vi "Examples.vi"(6 "Python version":string="3.9", 7 "Python":T1, 11 "Port":string) -> ()   [LabVIEW 2021]
uses:
  PythonCtrl.ctl
  Processors.ctl
  Comm_Global.vi
panel:
  out "Python files":string[](array[string])
  in  "Location":bool
  in  "Folder":u16(ring) items=["home"]
  in  "Files":i32(listbox)
  in  "Code":string="Loading..."
  in  "Paste":bool
  in  "Update":bool
  # "File Explorer\nversion 0"
  # "https://lego.github.io/MINDSTORMS-Robot-Inventor-hub-API/index.html"
  # "SPIKE Prime"
  # "Examples"
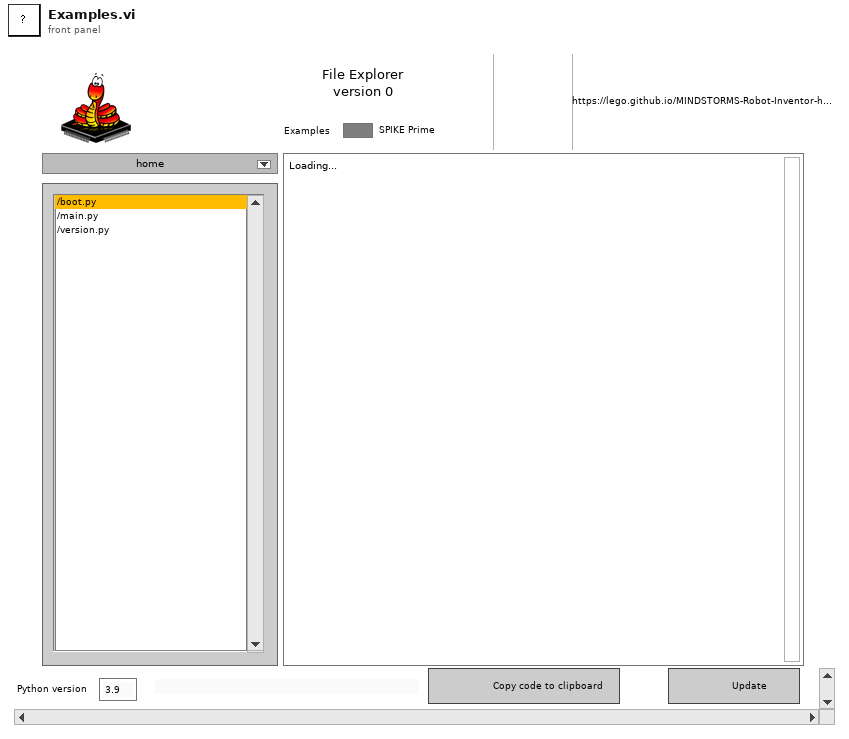
[diagram p1: front panel]
types:
  T1 = typedef "PythonCtrl.ctl" = cluster{"session":refnum<k35>, "PyPath":path, "Processor":T2, "Port":string, "version":string}
  T2 = typedef "Processors.ctl" = enum16{"SPIKE", "Pi", "Pi_ssh", "OpenMV", "Dunio"}
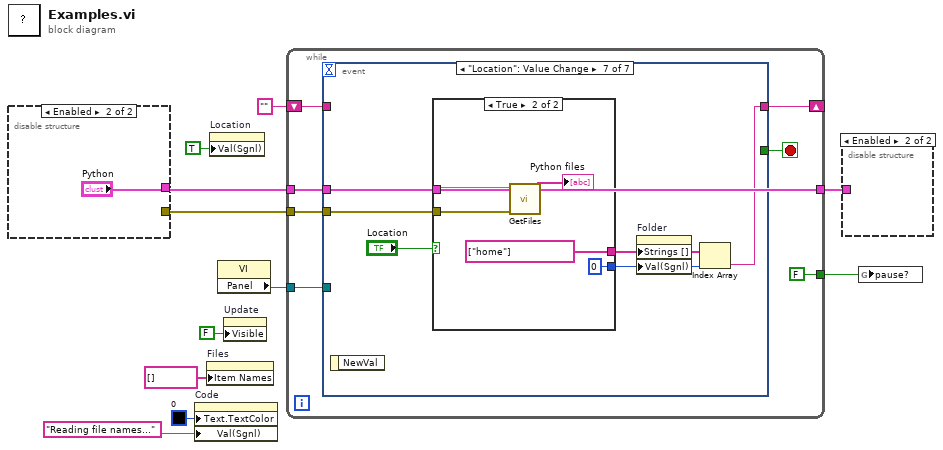
[diagram p0: block diagram]
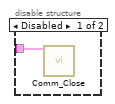
[diagram p2: hidden frame]
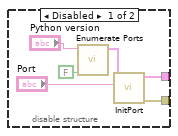
[diagram p3: hidden frame]
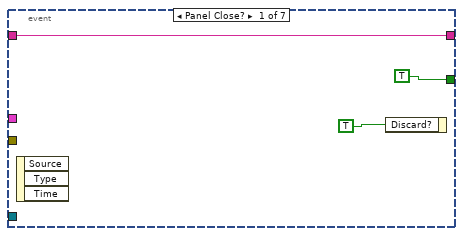
[diagram p4: hidden frame]
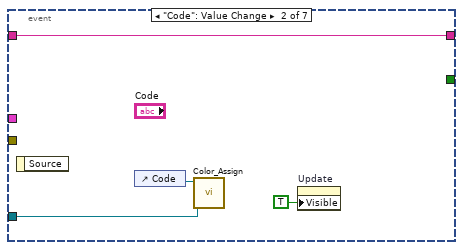
[diagram p5: hidden frame]
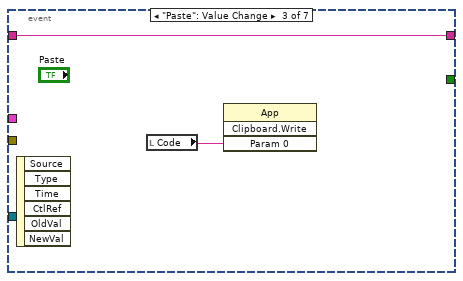
[diagram p6: hidden frame]
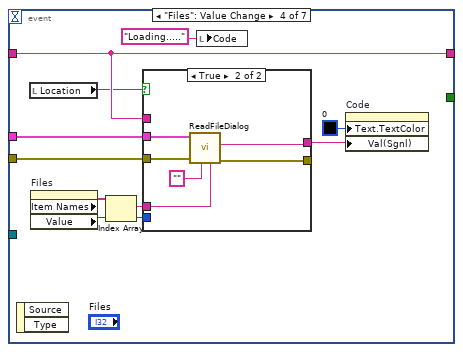
[diagram p7: hidden frame]
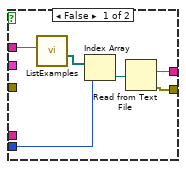
[diagram p8: hidden frame]
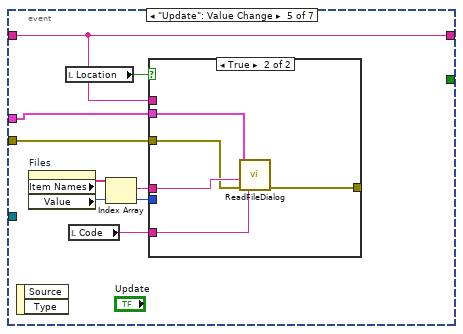
[diagram p9: hidden frame]
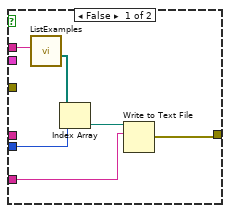
[diagram p10: hidden frame]
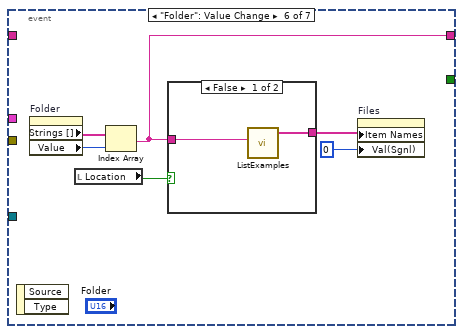
[diagram p11: hidden frame]
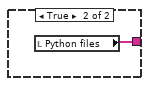
[diagram p12: hidden frame]
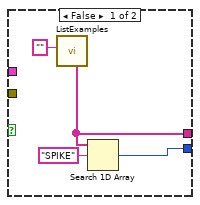
[diagram p13: hidden frame]
diagram:
  n1 = disable-structure shown="Enabled" {
    disable-tunnel: [w17 _] -> w5
    disable-tunnel: [w16 "Python"] -> w4
    frame Disabled {
      n2 = call "Enumerate Ports.vi"("list?"=FALSE, "Python version"="Python version") -> ("Python"=w14:T1)  [unwired: 5 in, 4 out]
      n3 = call "InitPort.vi"("Port"="Port", "Python"=w14) -> ("error out"=w17:errorcluster, "Python out"=w16:T1)  [unwired: 7 in, 1 out]
    }
    frame Enabled {
    }
  }
  n4 = property on="Code" class="Str"("Text.TextColor"=u32 0 ("Text.Text Colors:Text Color"), "Val(Sgnl)"="Reading file names...") -> ()  [unwired: 2 in, 2 out]
  n5 = property on="Files" class="LstBox (strict)"("Item Names"=string[] []) -> ()  [unwired: 2 in, 2 out]
  n6 = property on="Location" class="Bool (strict)"("Val(Sgnl)"=TRUE ("Value (Signaling)")) -> ()  [unwired: 2 in, 2 out]
  n7 = property class="VI"() -> ("Panel"=w11:refnum<vi>)  [unwired: 2 in, 2 out]
  n8 = property on="Update" class="Bool"("Visible"=FALSE) -> ()  [unwired: 2 in, 2 out]
  n9 = while {
    tunnel: w11 -> [w24]
    shift-right: [w23] -> _
    shift-left: "" ("Folder") -> [w22]
    tunnel: w4 -> [w19]
    tunnel: [FALSE ("pause?")] -> w7
    tunnel: w5 -> [w20]
    tunnel: [w19] -> w3
    stop <- w25 stop-if-true
    n10 = event shown="[6] \"Location\": Value Change" {
      selector: _ -> [_ _ _ _ _ _ _]
      dyn-events: _ -> [_ _ _ _ _ _ _]
      timeout: _ -> [_ _ _ _ _ _ _]
      tunnel: [TRUE ("stop") _ _ _ _ _ _] -> w25
      tunnel: w24 -> [_ w30 _ _ _ _ _]
      tunnel: [w26 w32 w34 w44 w64 w77 w88] -> w23
      tunnel: w22 -> [w26 w32 w34 w44 w64 _ _]
      tunnel: w19 -> [_ _ _ w42 w62 _ w90]
      tunnel: w20 -> [_ _ _ w37 w57 _ w85]
      event Panel Close? {
        n11 = event-data() -> ()  [unwired: 1 in, 3 out]
        n12 = event-data("Discard?"=TRUE ("stop")) -> ()  [unwired: 1 in, 1 out]
      }
      event "Code": Value Change {
        n13 = event-data() -> ()  [unwired: 1 in, 1 out]
        n14 = control-ref of="Code"() -> (w29:refnum<vi>)
        n15 = call "Color_Assign.vi"("Front Panel"=w30, "Code"=w29) -> ()  [unwired: 9 in, 1 out]
        n16 = property on="Update" class="Bool"("Visible"=TRUE) -> ()  [unwired: 2 in, 2 out]
      }
      event "Paste": Value Change {
        n17 = event-data() -> ()  [unwired: 1 in, 6 out]
        n18 = local read "Code"() -> (w33:string)
        n19 = invoke class="App" method="Clipboard.Write"("Param 0"=w33) -> ()  [unwired: 3 in, 4 out]
      }
      event "Files": Value Change {
        n20 = event-data() -> ()  [unwired: 1 in, 2 out]
        n21 = local read "Location"() -> (w43:bool)
        n22 = property on="Files" class="LstBox (strict)"() -> ("Item Names"=w41:string[], "Value"=w39:i32)  [unwired: 2 in, 2 out]
        n23 = Index Array(array=w41, index=w39) -> (element=w40:string)
        n24 = case shown="True" w43 {
          tunnel: [w48 w55] -> w36
          tunnel: w44 -> [w47 _]
          tunnel: [w46 w54] -> _
          tunnel: w42 -> [_ w51]
          tunnel: w40 -> [_ w53]
          tunnel: w39 -> [w45 _]
          tunnel: w37 -> [_ w52]
          frame False {
            n25 = call "ListExamples.vi"("Folder"=w47) -> ("Paths"=w50:path[])  [unwired: 6 in, 4 out]
            n26 = Index Array(array=w50, index=w45) -> (element=w49:path)
            n27 = Read from Text File(file (use dialog)=w49) -> (text=w48:string, error out=w46:errorcluster)  [unwired: 3 in, 2 out]
          }
          frame True {
            n28 = call "ReadFileDialog.vi"("File Text"="" ("Folder"), "error in (no error)"=w52, "File name"=w53, "Python in"=w51) -> ("error out"=w54:errorcluster, "Console"=w55:string)  [unwired: 6 in]
          }
        }
        n29 = local write "Code"("Loading....." ("Folder")) -> ()
        n30 = property on="Code" class="Str"("Text.TextColor"=u32 0 ("Text.Text Colors:Text Color"), "Val(Sgnl)"=w36) -> ()  [unwired: 2 in, 2 out]
      }
      event "Update": Value Change {
        n31 = event-data() -> ()  [unwired: 1 in, 2 out]
        n32 = property on="Files" class="LstBox (strict)"() -> ("Item Names"=w61:string[], "Value"=w59:i32)  [unwired: 2 in, 2 out]
        n33 = local read "Location"() -> (w63:bool)
        n34 = local read "Code"() -> (w58:string)
        n35 = Index Array(array=w61, index=w59) -> (element=w60:string)
        n36 = case shown="True" w63 {
          tunnel: w64 -> [w68 _]
          tunnel: [w67 w75] -> _
          tunnel: w62 -> [_ w72]
          tunnel: w60 -> [_ w74]
          tunnel: w59 -> [w66 _]
          tunnel: w58 -> [w65 w73]
          tunnel: w57 -> [_ w71]
          frame False {
            n37 = call "ListExamples.vi"("Folder"=w68) -> ("Paths"=w70:path[])  [unwired: 6 in, 4 out]
            n38 = Index Array(array=w70, index=w66) -> (element=w69:path)
            n39 = Write to Text File(file (use dialog)=w69, text=w65) -> (error out=w67:errorcluster)  [unwired: 2 in, 2 out]
          }
          frame True {
            n40 = call "ReadFileDialog.vi"("File Text"=w73, "error in (no error)"=w71, "File name"=w74, "Python in"=w72) -> ("error out"=w75:errorcluster)  [unwired: 6 in, 1 out]
          }
        }
      }
      event "Folder": Value Change {
        n41 = event-data() -> ()  [unwired: 1 in, 2 out]
        n42 = property on="Folder" class="Ring (strict)"() -> ("Strings []"=w81:string[], "Value"=w80:u16)  [unwired: 2 in, 2 out]
        n43 = local read "Location"() -> (w76:bool)
        n44 = Index Array(array=w81, index=w80) -> (element=w77:string)
        n45 = case shown="False" w76 {
          tunnel: [w83 w84] -> w79
          tunnel: w77 -> [w82 _]
          frame False {
            n46 = call "ListExamples.vi"("Folder"=w82) -> ("filenames"=w83:string[])  [unwired: 6 in, 4 out]
          }
          frame True {
            n47 = local read "Python files"() -> (w84:string[])
          }
        }
        n48 = property on="Files" class="LstBox (strict)"("Item Names"=w79, "Val(Sgnl)"=u16 0 ("Value (Signaling)")) -> ()  [unwired: 2 in, 2 out]
      }
      event "Location": Value Change {
        n49 = event-data() -> ()  [unwired: 1 in, 1 out]
        n50 = case shown="True" "Location" {
          tunnel: w90 -> [_ w95]
          tunnel: [w93 string[] ["home"] ("folder names")] -> w87
          tunnel: [w91 u16 0 ("Value (Signaling)")] -> w86
          tunnel: w85 -> [_ w96]
          frame False {
            n51 = call "ListExamples.vi"("Folder"="") -> ("folder names"=w93:string[])  [unwired: 6 in, 4 out]
            n52 = Search 1D Array(1D array=w93, element="SPIKE") -> (index of element=w91:i32)  [unwired: 1 in]
          }
          frame True {
            n53 = call "GetFiles.vi"("error in (no error)"=w96, "Python"=w95) -> ("all files"=→"Python files":string[])  [unwired: 8 in, 1 out]
          }
        }
        n54 = property on="Folder" class="Ring (strict)"("Strings []"=w87, "Val(Sgnl)"=w86) -> ()  [unwired: 2 in, 2 out]
        n55 = Index Array(array=w87, index=w86) -> (element=w88:string)
      }
    }
  }
  n56 = disable-structure shown="Enabled" {
    disable-tunnel: w3 -> [w100 _]
    frame Disabled {
      n57 = call "Comm_Close.vi"("Python in"=w100) -> ()  [unwired: 9 in, 2 out]
    }
    frame Enabled {
    }
  }
  n58 = global write "Comm_Global.vi" "pause?"(w7) -> ()
